vi "GetReportSelection(SubVI).vi"(8 "error in (no error)":errorcluster, 11 "ListBox in":refnum<vi>) -> (0 "error out":errorcluster, 3 "Selected Report":string)   [LabVIEW 2017, in "MainFrameLib.lvlib"]
uses:
  MainFrameLib.lvlib
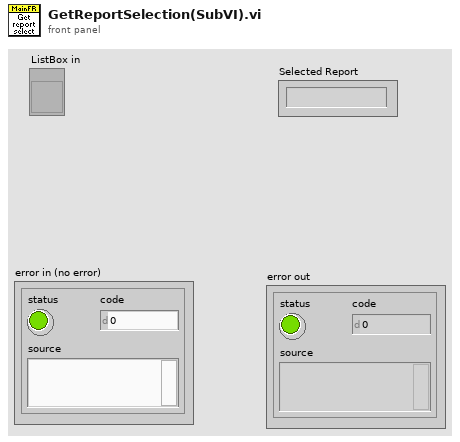
[diagram p1: front panel]
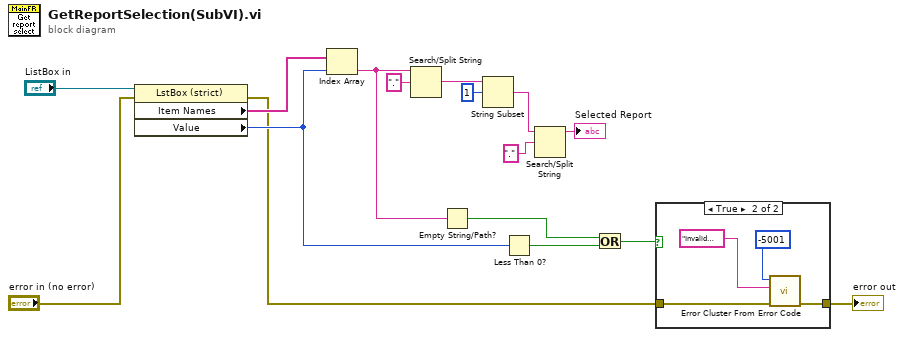
[diagram p0: block diagram]
diagram:
  n1 = property class="LstBox (strict)"(reference="ListBox in", error in="error in (no error)") -> (error out=w1:errorcluster, "Item Names"=w8:string[], "Value"=w7:i32)  [unwired: 1 out]
  n2 = Index Array(array=w8, index=w7) -> (element=w6:string)
  n3 = Search/Split String(string=w6, search string/char (-)=".") -> (match + rest of string=w12:string)  [unwired: 1 in, 2 out]
  n4 = Empty String/Path?(string/path=w6) -> (empty?=w5:bool)
  n5 = String Subset(string=w12, offset (0)=1) -> (substring=w13:string)  [unwired: 1 in]
  n6 = Less Than 0?(x=w7) -> (x < 0?=w9:bool)
  n7 = Search/Split String(string=w13, search string/char (-)=".") -> (substring before match=→"Selected Report":string)  [unwired: 1 in, 2 out]
  n8 = Or(x=w5, y=w9) -> (x .or. y?=w3:bool)
  n9 = case shown="True" w3 {
    tunnel: w1 -> [w17 w21]
    tunnel: [w17 w20] -> w2
    frame False {
    }
    frame True {
      n10 = call <vilib>:"Error Cluster From Error Code.vi"("error in (no error)"=w21, "error message (\"\")"="Invalid report selection " ("error message (\"\")"), "error code (0)"=-5001) -> ("error out"=w20:errorcluster)  [unwired: 6 in]
    }
  }
  "error out" <- w2
